vi "o3 TCP Packet.vi"(0 "ID":string, 5 "Version":string, 7 "utc_time":u32, 9 "PTP Sync":string="0", 11 "ue9LJ temp":u16, 12 "Flight Number":string, 13 "Data Array":string[](array[string])) -> (8 "TCP Binary Packet":string)   [LabVIEW 2014]
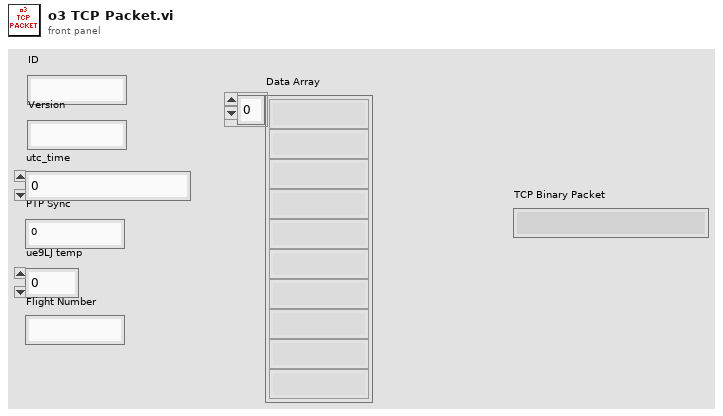
[diagram p1: front panel]
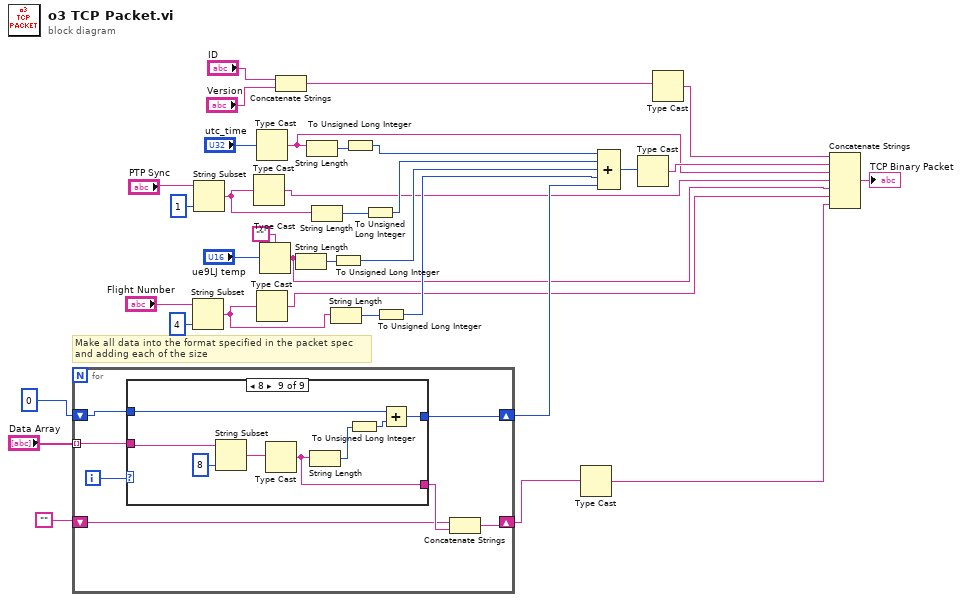
[diagram p0: block diagram]
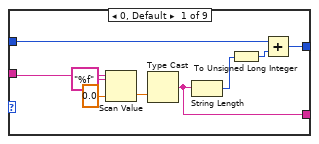
[diagram p2: hidden frame]
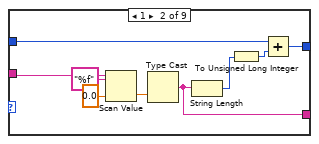
[diagram p3: hidden frame]
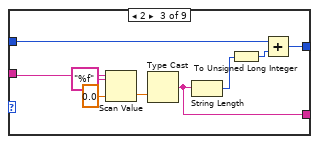
[diagram p4: hidden frame]
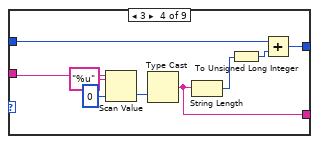
[diagram p5: hidden frame]
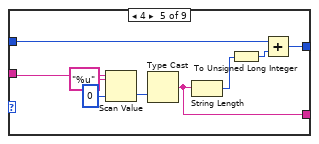
[diagram p6: hidden frame]
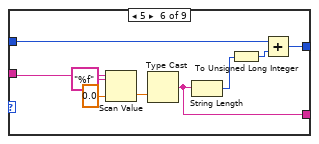
[diagram p7: hidden frame]
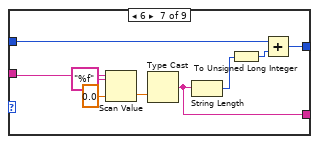
[diagram p8: hidden frame]
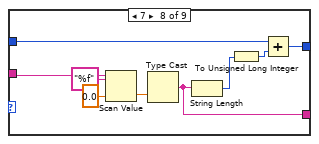
[diagram p9: hidden frame]
diagram:
  # "Make all data into the format specified in the packet spec\nand adding each of the size"
  n1 = for {
    tunnel: "Data Array" -> [w40] mode=indexing
    shift-right: [w38] -> w14
    shift-left: u32 0 -> [w39]
    shift-right: [w37] -> w1
    shift-left: "" -> [w35]
    i -> [w41]
    n2 = case shown="8" w41 {
      tunnel: w40 -> [w48 w57 w66 w75 w84 w93 w102 w111 w115]
      tunnel: w39 -> [w46 w55 w64 w73 w82 w91 w100 w109 w121]
      tunnel: [w43 w52 w61 w70 w79 w88 w97 w106 w118] -> w38
      tunnel: [w42 w51 w60 w69 w78 w87 w96 w105 w117] -> w36
      frame 0, Default {
        n3 = Scan Value(string=w48, format string="%f", default (0 dbl)=sgl 0.0 ("default (0 I32)")) -> (value=w50:sgl)  [unwired: 1 out]
        n4 = Type Cast(x=w50) -> (*(type *) &x=w42:string)  [unwired: 1 in]
        n5 = String Length(string=w42) -> (length=w45:i32)
        n6 = To Unsigned Long Integer(number=w45) -> (unsigned 32bit integer=w44:u32)
        n7 = Add(x=w46, y=w44) -> (x+y=w43:u32)
      }
      frame 1 {
        n8 = Scan Value(string=w57, format string="%f", default (0 dbl)=sgl 0.0 ("default (0 I32)")) -> (value=w59:sgl)  [unwired: 1 out]
        n9 = Type Cast(x=w59) -> (*(type *) &x=w51:string)  [unwired: 1 in]
        n10 = String Length(string=w51) -> (length=w54:i32)
        n11 = To Unsigned Long Integer(number=w54) -> (unsigned 32bit integer=w53:u32)
        n12 = Add(x=w55, y=w53) -> (x+y=w52:u32)
      }
      frame 2 {
        n13 = Scan Value(string=w66, format string="%f", default (0 dbl)=sgl 0.0 ("default (0 I32)")) -> (value=w68:sgl)  [unwired: 1 out]
        n14 = Type Cast(x=w68) -> (*(type *) &x=w60:string)  [unwired: 1 in]
        n15 = String Length(string=w60) -> (length=w63:i32)
        n16 = To Unsigned Long Integer(number=w63) -> (unsigned 32bit integer=w62:u32)
        n17 = Add(x=w64, y=w62) -> (x+y=w61:u32)
      }
      frame 3 {
        n18 = Scan Value(string=w75, format string="%u", default (0 dbl)=u16 0 ("default (0 I32)")) -> (value=w77:u16)  [unwired: 1 out]
        n19 = Type Cast(x=w77) -> (*(type *) &x=w69:string)  [unwired: 1 in]
        n20 = String Length(string=w69) -> (length=w72:i32)
        n21 = To Unsigned Long Integer(number=w72) -> (unsigned 32bit integer=w71:u32)
        n22 = Add(x=w73, y=w71) -> (x+y=w70:u32)
      }
      frame 4 {
        n23 = Scan Value(string=w84, format string="%u", default (0 dbl)=u16 0 ("default (0 I32)")) -> (value=w86:u16)  [unwired: 1 out]
        n24 = Type Cast(x=w86) -> (*(type *) &x=w78:string)  [unwired: 1 in]
        n25 = String Length(string=w78) -> (length=w81:i32)
        n26 = To Unsigned Long Integer(number=w81) -> (unsigned 32bit integer=w80:u32)
        n27 = Add(x=w82, y=w80) -> (x+y=w79:u32)
      }
      frame 5 {
        n28 = Scan Value(string=w93, format string="%f", default (0 dbl)=sgl 0.0 ("default (0 I32)")) -> (value=w95:sgl)  [unwired: 1 out]
        n29 = Type Cast(x=w95) -> (*(type *) &x=w87:string)  [unwired: 1 in]
        n30 = String Length(string=w87) -> (length=w90:i32)
        n31 = To Unsigned Long Integer(number=w90) -> (unsigned 32bit integer=w89:u32)
        n32 = Add(x=w91, y=w89) -> (x+y=w88:u32)
      }
      frame 6 {
        n33 = Scan Value(string=w102, format string="%f", default (0 dbl)=sgl 0.0 ("default (0 I32)")) -> (value=w104:sgl)  [unwired: 1 out]
        n34 = Type Cast(x=w104) -> (*(type *) &x=w96:string)  [unwired: 1 in]
        n35 = String Length(string=w96) -> (length=w99:i32)
        n36 = To Unsigned Long Integer(number=w99) -> (unsigned 32bit integer=w98:u32)
        n37 = Add(x=w100, y=w98) -> (x+y=w97:u32)
      }
      frame 7 {
        n38 = Scan Value(string=w111, format string="%f", default (0 dbl)=sgl 0.0 ("default (0 I32)")) -> (value=w113:sgl)  [unwired: 1 out]
        n39 = Type Cast(x=w113) -> (*(type *) &x=w105:string)  [unwired: 1 in]
        n40 = String Length(string=w105) -> (length=w108:i32)
        n41 = To Unsigned Long Integer(number=w108) -> (unsigned 32bit integer=w107:u32)
        n42 = Add(x=w109, y=w107) -> (x+y=w106:u32)
      }
      frame 8 {
        n43 = String Subset(string=w115, length (rest)=8 ("length (rest)")) -> (substring=w114:string)  [unwired: 1 in]
        n44 = Type Cast(x=w114) -> (*(type *) &x=w117:string)  [unwired: 1 in]
        n45 = String Length(string=w117) -> (length=w120:i32)
        n46 = To Unsigned Long Integer(number=w120) -> (unsigned 32bit integer=w119:u32)
        n47 = Add(x=w121, y=w119) -> (x+y=w118:u32)
      }
    }
    n48 = Concatenate Strings(w35, w36) -> (w37:string)
  }
  n49 = String Subset(string="Flight Number", length (rest)=4 ("length (rest)")) -> (substring=w5:string)  [unwired: 1 in]
  n50 = String Subset(string="PTP Sync", length (rest)=1 ("length (rest)")) -> (substring=w9:string)  [unwired: 1 in]
  n51 = Type Cast(x=w9) -> (*(type *) &x=w8:string)  [unwired: 1 in]
  n52 = Type Cast(x="utc_time") -> (*(type *) &x=w10:string)  [unwired: 1 in]
  n53 = Type Cast(x=w5) -> (*(type *) &x=w6:string)  [unwired: 1 in]
  n54 = Type Cast(type="", x="ue9LJ temp") -> (*(type *) &x=w7:string)
  n55 = Concatenate Strings("ID", "Version") -> (w32:string)
  n56 = String Length(string=w7) -> (length=w23:i32)
  n57 = String Length(string=w10) -> (length=w31:i32)
  n58 = String Length(string=w9) -> (length=w27:i32)
  n59 = String Length(string=w5) -> (length=w19:i32)
  n60 = To Unsigned Long Integer(number=w23) -> (unsigned 32bit integer=w21:u32)
  n61 = To Unsigned Long Integer(number=w31) -> (unsigned 32bit integer=w29:u32)
  n62 = To Unsigned Long Integer(number=w27) -> (unsigned 32bit integer=w25:u32)
  n63 = To Unsigned Long Integer(number=w19) -> (unsigned 32bit integer=w17:u32)
  n64 = Type Cast(x=w1) -> (*(type *) &x=w4:string)  [unwired: 1 in]
  n65 = Compound Arithmetic op=ADD(w29, w25, w21, w17, w14) -> (w12:u32)
  n66 = Type Cast(x=w12) -> (*(type *) &x=w11:string)  [unwired: 1 in]
  n67 = Type Cast(x=w32) -> (*(type *) &x=w13:string)  [unwired: 1 in]
  n68 = Concatenate Strings(w13, w11, w10, w8, w7, w6, w4) -> (→"TCP Binary Packet":string)
